vi "Result.Parse Test Utility Rtn Data, Code, StdErr, StdOut, Create Result Data_V3.vi"(7 "Name":string, 8 "BaseCode":i32, 9 "RtnCode":i32, 10 "StdErr":string, 11 "StdOut":string) -> (3 "RTN Data":T1 {"MeasData"."Status" items=["LOG", "PASS", "FAIL", "ERROR"]; "Attr"."Status" items=["LOG", "PASS", "FAIL", "ERROR"]; "Num"."Status" items=["LOG", "PASS", "FAIL", "ERROR"]})   [LabVIEW 2018]
uses:
  TestExec/TestExec.Local Result Data.ctl
  Result.Attribute.ctl
  Result.Measurement and Attribute Item Status.ctl
  Result.Numeric.ctl
  Result.Limit Type.ctl
  Result XML/TestResult.SW Item.ctl
  Reports/Report.Result FileDataObject.ctl
  Result.Measurement Item.ctl
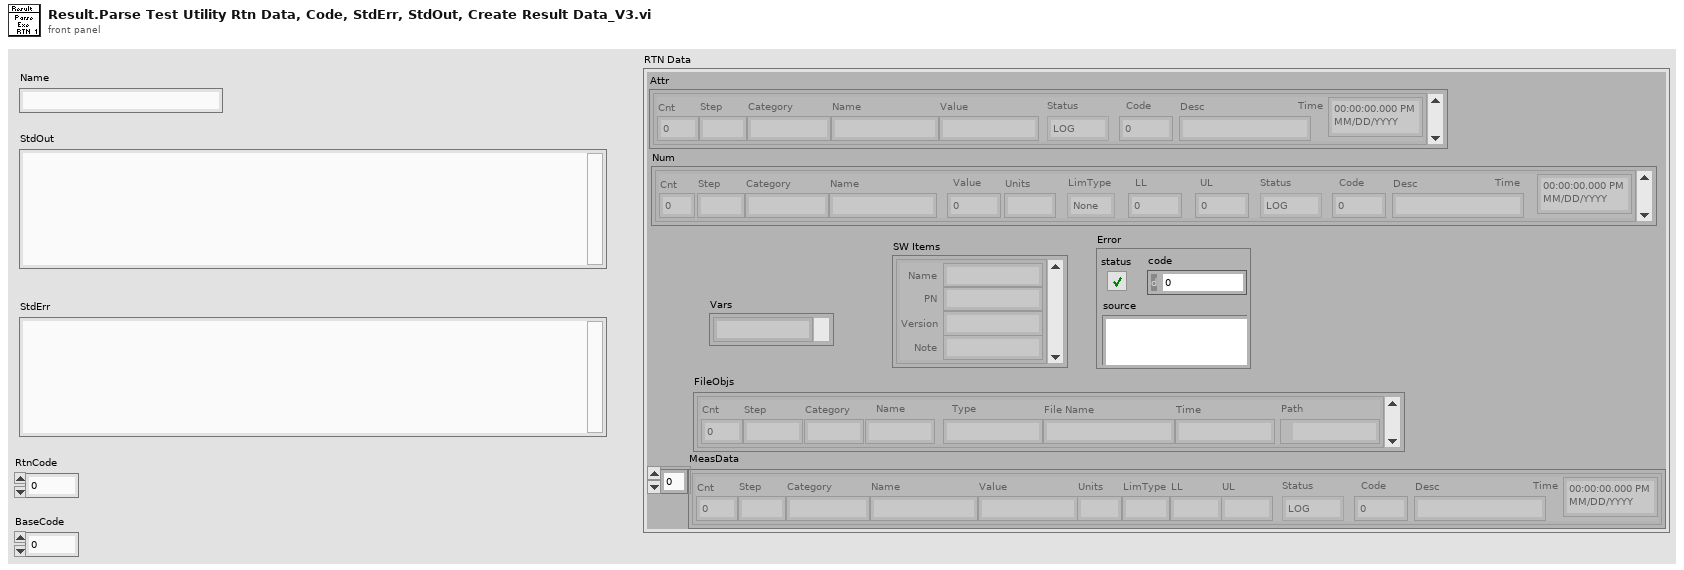
[diagram p1: front panel]
types:
  T1 = typedef "TestExec.Local Result Data.ctl" = cluster{"Attr":T2[], "Num":T4[], "UUT Props":string[][], "Vars":string[][], "SW Items":T6[], "Error":errorcluster, "Step":i32, "FileObjs":T7[], "MeasData":T8[]}
  T2 = typedef "Result.Attribute.ctl" = cluster{"Cnt":i32, "Step":string, "Category":string, "Name":string, "Value":string, "Status":T3, "Code":i32, "Desc":string, "Time":timestamp}
  T3 = typedef "Result.Measurement and Attribute Item Status.ctl" = i32
  T4 = typedef "Result.Numeric.ctl" = cluster{"Cnt":i32, "Step":string, "Category":string, "Name":string, "Value":dbl, "Units":string, "LimType":T5, "LL":dbl, "UL":dbl, "Status":T3, "Code":i32, "Desc":string, "Time":timestamp}
  T5 = typedef "Result.Limit Type.ctl" = enum16{"None", "EQ", "NE", "GT", "LT", "GE", "LE", "GTLT", "GELE", "GELT", "GTLE", "LTGT", "LEGE", "LEGT", "LTGE", "Contains", "NotContains"}
  T6 = typedef "TestResult.SW Item.ctl" = cluster{"Name":string, "PN":string, "Version":string, "Note":string}
  T7 = typedef "Report.Result FileDataObject.ctl" = cluster{"Cnt":i32, "Step":string, "Category":string, "Name":string, "Type":string, "File Name":string, "Time":string, "Path":path}
  T8 = typedef "Result.Measurement Item.ctl" = cluster{"Cnt":i32, "Step":string, "Category":string, "Name":string, "Value":string, "Units":string, "LimType":string, "LL":string, "UL":string, "Status":T3, "Code":i32, "Desc":string, "Time":timestamp}
  T9 = cluster{"Name":string, "RTN Data":T1, "StdOut":string, "StdErr":string, "BaseCode":i32, "RtnCode":i32}
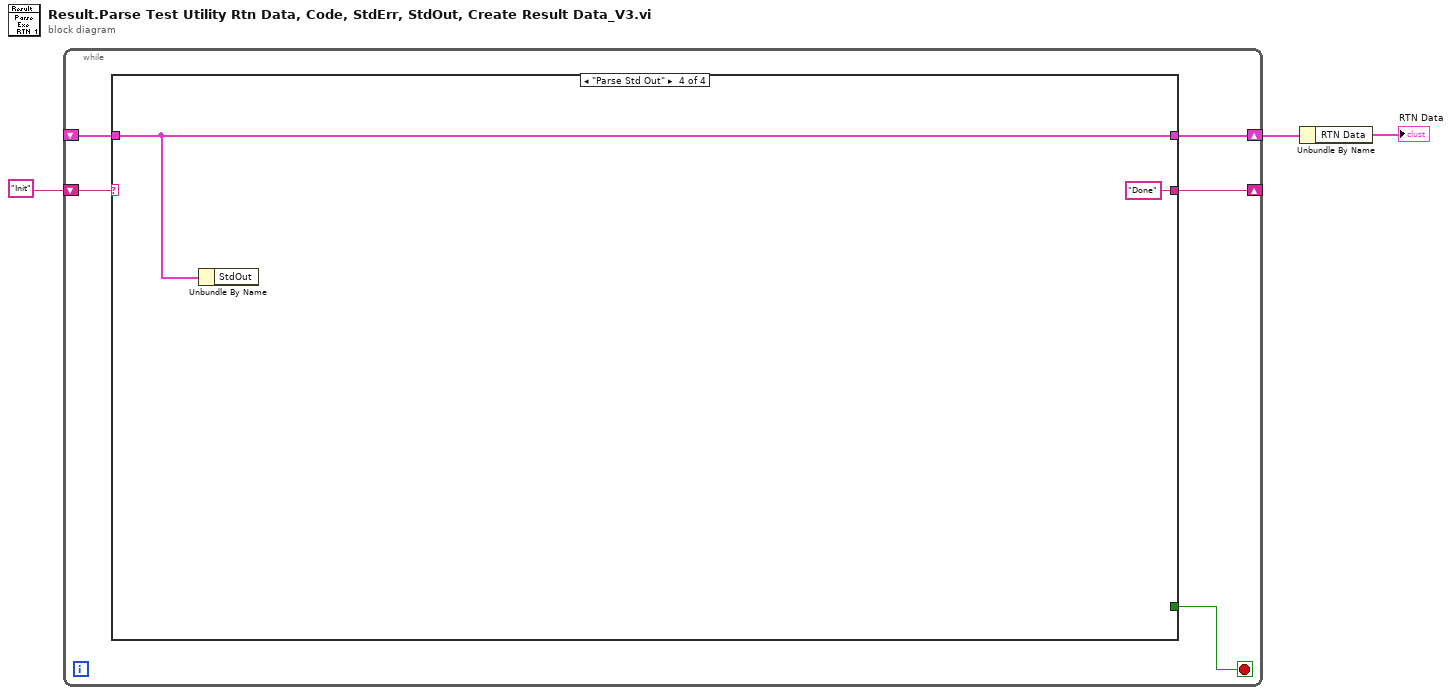
[diagram p0: block diagram]
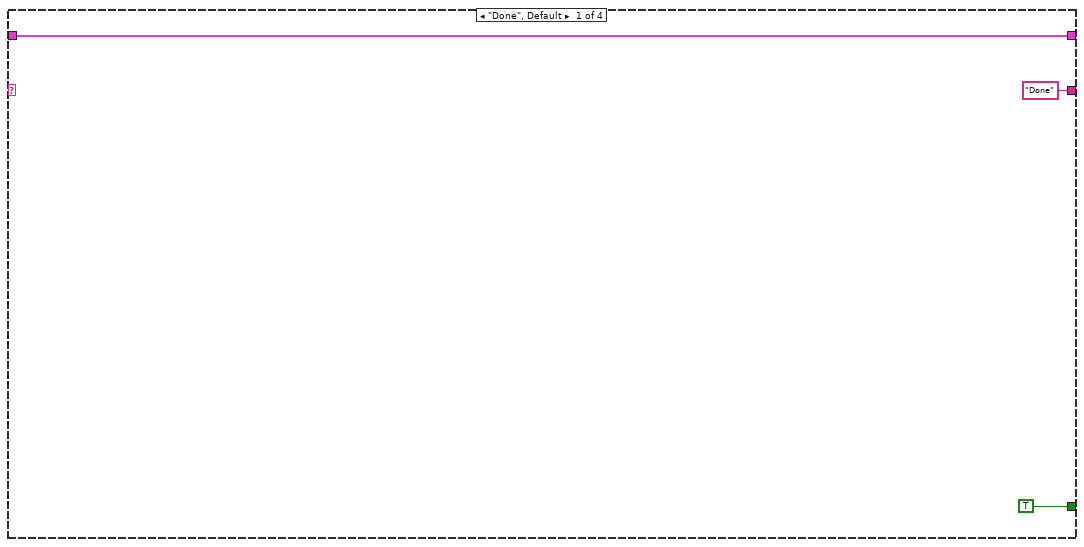
[diagram p2: hidden frame]
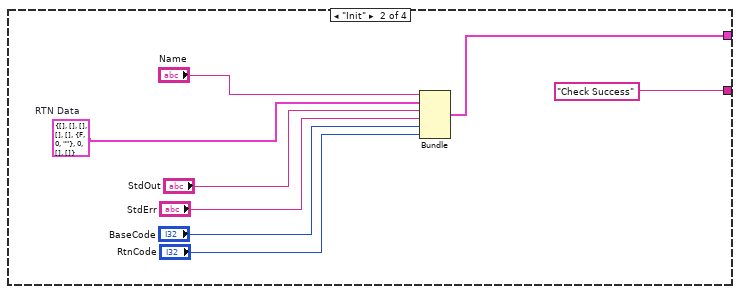
[diagram p3: hidden frame]
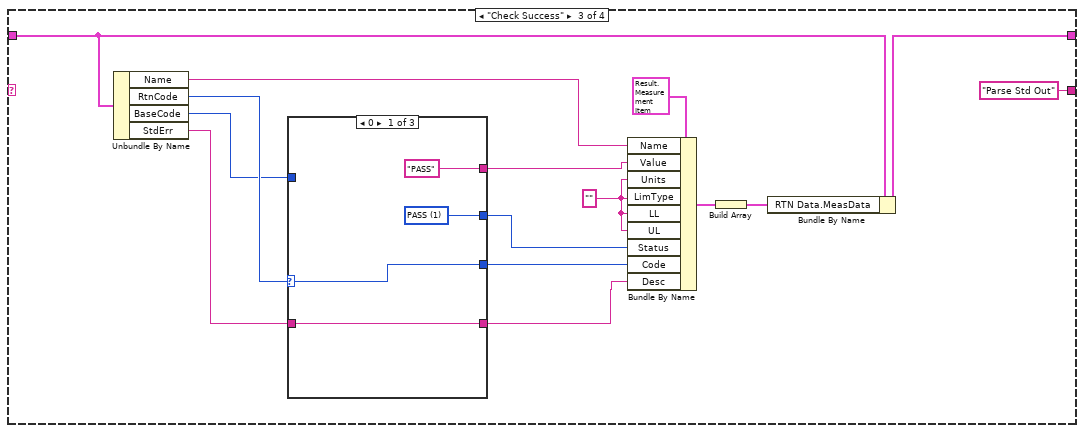
[diagram p4: hidden frame]
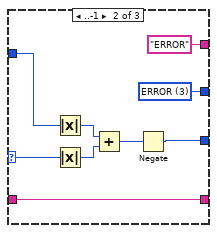
[diagram p5: hidden frame]
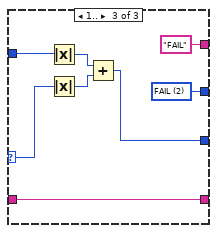
[diagram p6: hidden frame]
diagram:
  n1 = while {
    shift-right: [w5] -> _
    shift-left: "Init" -> [w8]
    shift-right: [w6] -> w2
    shift-left: _ -> [w7]
    stop <- w4 stop-if-true
    n2 = case shown="\"Parse Std Out\"" w8 {
      tunnel: w7 -> [w11 _ w21 w56]
      tunnel: [w11 w15 w22 w56] -> w6
      tunnel: ["Done" "Check Success" "Parse Std Out" "Done"] -> w5
      tunnel: [TRUE _ _ _] -> w4
      frame "Done", Default {
      }
      frame "Init" {
        w12 = T1 {"Attr"=[], "Num"=[], "UUT Props"=[], "Vars"=[], "SW Items"=[], "Error"={"status"=FALSE, "code"=0, "source"=""}, "Step"=0, "FileObjs"=[], "MeasData"=[]}  # RTN Data
        n3 = Bundle("Name"="Name", "RTN Data"=w12, "StdOut"="StdOut", "StdErr"="StdErr", "BaseCode"="BaseCode", "RtnCode"="RtnCode") -> (w15:T9)  [unwired: 1 in]
      }
      frame "Check Success" {
        w28 = ""
        n4 = Unbundle By Name(w21) -> ("Name"=w27:string, "RtnCode"=w26:i32, "BaseCode"=w25:i32, "StdErr"=w24:string)
        n5 = case shown="0" w26 {
          selector: w26 -> [w36 w45 w50]
          tunnel: [w38 w47 w55] -> w31
          tunnel: ["PASS" "ERROR" "FAIL"] -> w32
          tunnel: w25 -> [_ w44 w51]
          tunnel: [w36 w40 w49] -> w33
          tunnel: w24 -> [w35 w39 w48]
          tunnel: [w35 w39 w48] -> w34
          frame 0 {
            w38 = T3 1 items=["LOG", "PASS", "FAIL", "ERROR"] ("Status")
          }
          frame ..-1 {
            w47 = T3 3 items=["LOG", "PASS", "FAIL", "ERROR"] ("Status")
            n6 = Absolute Value(x=w44) -> (abs(x)=w43:i32)
            n7 = Absolute Value(x=w45) -> (abs(x)=w42:i32)
            n8 = Add(x=w43, y=w42) -> (x+y=w41:i32)
            n9 = Negate(x=w41) -> (-x=w40:i32)
          }
          frame 1.. {
            w55 = T3 2 items=["LOG", "PASS", "FAIL", "ERROR"] ("Status")
            n10 = Absolute Value(x=w51) -> (abs(x)=w53:i32)
            n11 = Absolute Value(x=w50) -> (abs(x)=w52:i32)
            n12 = Add(x=w53, y=w52) -> (x+y=w49:i32)
          }
        }
        n13 = Bundle By Name(cluster=T8 {"Cnt"=0, "Step"="", "Category"="", "Name"="", "Value"="", "Units"="", "LimType"="", "LL"="", "UL"="", "Status"=0, "Code"=0, "Desc"="", "Time"=timestamp(0 s since 1904-01-01)} ("Meas"), "Name"=w27, "Value"=w32, "Units"=w28, "LimType"=w28, "LL"=w28, "UL"=w28, "Status"=w31, "Code"=w33, "Desc"=w34) -> (w30:T8)
        n14 = Build Array(w30) -> (w23:T8[])
        n15 = Bundle By Name(cluster=w21, "RTN Data.MeasData"=w23) -> (w22:T9)
      }
      frame "Parse Std Out" {
        n16 = Unbundle By Name(w56) -> ()  [unwired: 1 out]
      }
    }
  }
  n17 = Unbundle By Name(w2) -> ("RTN Data"=→"RTN Data":T1)
